vi "Read Laser State.vi"(8 "error in (no error)":errorcluster, 11 "Laser State Data in":refnum<class "Laser State Data.lvclass">) -> (0 "error out":errorcluster, 2 "Laser State":T1, 3 "Laser State Data out":refnum<class "Laser State Data.lvclass">)   [LabVIEW 2022 SP3, in "Laser State Data.lvclass"]
uses:
  Laser State Data.lvclass
  Laser State Data.lvclass/Laser State Data.ctl
  Laser State.ctl
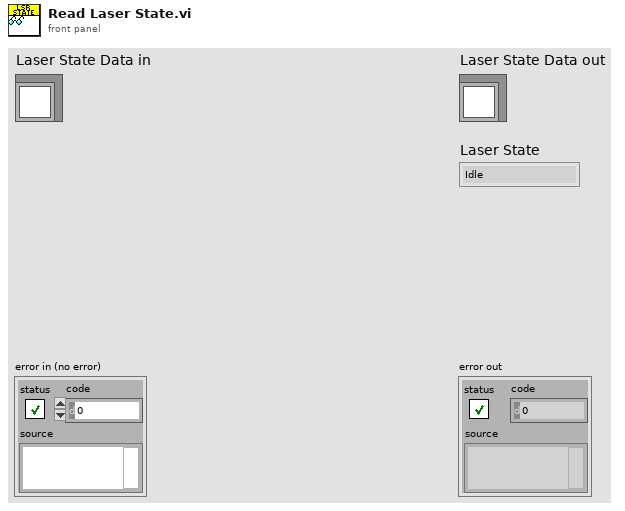
[diagram p1: front panel]
types:
  T1 = typedef "Laser State Data.lvclass/Laser State.ctl" = enum16{"Idle", "Warming", "Ready", "Firing"}
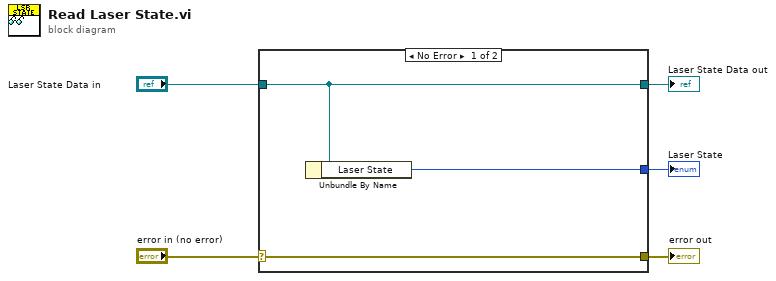
[diagram p0: block diagram]
diagram:
  n1 = case shown="No Error" "error in (no error)" {
    selector: "error in (no error)" -> [w8 w9]
    tunnel: [w8 w9] -> w4
    tunnel: [w7 w10] -> w2
    tunnel: "Laser State Data in" -> [w7 w10]
    tunnel: [w6 _] -> w1
    frame No Error {
      n2 = Unbundle By Name(w7) -> ("Laser State"=w6:T1)
    }
    frame Error {
    }
  }
  "error out" <- w4
  "Laser State Data out" <- w2
  "Laser State" <- w1
